vi "RTMain.Close.vi"(11 "cluster":T1 {"Parameters"."Settings"."Data Refs"."Write Refs" format="%.0x"; "Parameters"."Settings"."Data Refs"."Read Refs" format="%.0x"; "Parameters"."Settings"."Write Locations"."DataType" items=["Boolean"=1, "SByte"=2, "Byte"=3, "Int16"=4, "UInt16"=5, "Int32"=6, "UInt32"=7, "Int64"=8, "UInt64"=9, "Float"=10, "Double"=11, "String"=12, "DateTime"=13, "ByteString"=15, "Array of Boolean"=101, "Array of SByte"=102, "Array of Byte"=103, "Array of Int16"=104, "Array of UInt16"=105, "Array of Int32"=106, "Array of UInt32"=107, "Array of Int64"=108, "Array of UInt64"=109, "Array of Float"=110, "Array of Double"=111, "Array of String"=112, "Array of DateTime"=113, "Array of ByteString"=115]}) -> ()   [LabVIEW 2015, in "OPC UA Client Engine.lvlib"]
uses:
  OPC UA Client Engine.lvlib
  Types/Main.StateVariables.ctl
  <vilib>/NI/NIVS Inline Async API/_VS Inline Async API/VS Inline Async API/VS Inline Async API.lvclass
  Types/Poll.Parameters.ctl
  Shared/Compiled.Settings.ctl
  Shared/OPCConnection.Properties.ctl
  Shared/Poll.ListProperties.ctl
  Shared/Tag.WriteProperties.Info.ctl
  Shared/Tags.ReadWriteRefs.ctl
  <vilib>/NI Veristand/Custom Device API/Data Reference.ctl
  <vilib>/NI Veristand/Custom Device API/Custom Device Target Type.ctl
  <vilib>/NI Veristand/Custom Device Tools/Custom Device Utility Library/Custom Device Utility Library.lvlib
  Shared/OPC UA Client Shared.lvlib
  <vilib>/NI VeriStand/Custom Device API/Custom Device API.lvlib
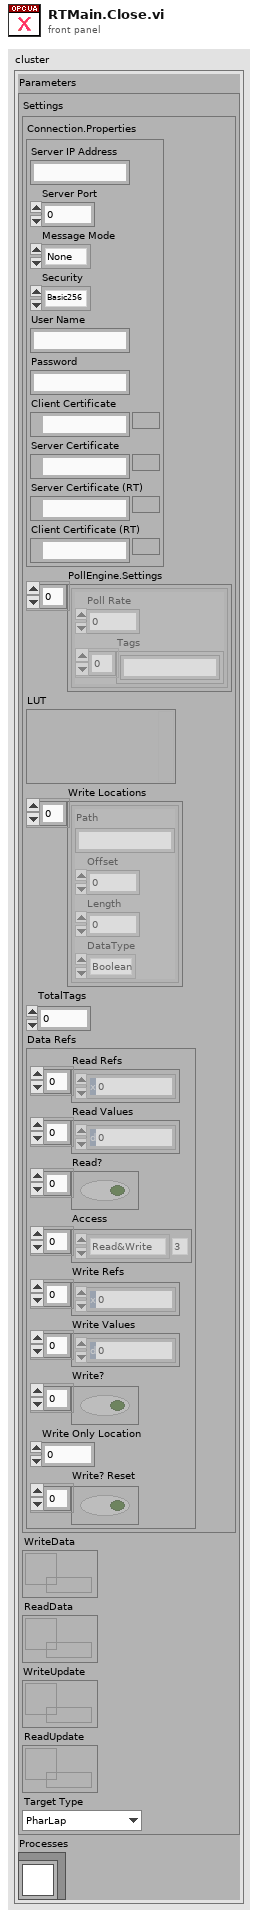
[diagram p1: front panel]
types:
  T1 = typedef "OPC UA Client Engine.lvlib/Main.StateVariables.ctl" = cluster{"Parameters":T2, "Processes":refnum<class "VS Inline Async API.lvclass">}
  T2 = typedef "OPC UA Client Engine.lvlib/Poll.Parameters.ctl" = cluster{"Settings":T3, "WriteData":refnum<k33>, "ReadData":refnum<k33>, "WriteUpdate":refnum<k33>, "ReadUpdate":refnum<k33>, "Target Type":T9}
  T3 = typedef "OPC UA Client Shared.lvlib/Compiled.Settings.ctl" = cluster{"Connection.Properties":T4, "PollEngine.Settings":T5[], "LUT":variant, "Write Locations":T6[], "TotalTags":u32, "Data Refs":T7}
  T4 = typedef "OPC UA Client Shared.lvlib/OPCConnection.Properties.ctl" = cluster{"Server IP Address":string, "Server Port":u16, "Message Mode":enum16{"None", "Sign", "Sign and Encrypt"}, "Security":enum16{"Basic256", "Basic128Rsa15"}, "User Name":string, "Password":string, "Client Certificate":path, "Server Certificate":path, "Server Certificate (RT)":path, "Client Certificate (RT)":path}
  T5 = typedef "OPC UA Client Shared.lvlib/Poll.ListProperties.ctl" = cluster{"Poll Rate":dbl, "Tags":string[]}
  T6 = typedef "OPC UA Client Shared.lvlib/Tag.WriteProperties.Info.ctl" = cluster{"Path":string, "Offset":i32, "Length":i32, "DataType":u32}
  T7 = typedef "OPC UA Client Shared.lvlib/Tags.ReadWriteRefs.ctl" = cluster{"Read Refs":T8[], "Read Values":dbl[], "Read?":bool[], "Access":enum8{"Null", "Read", "Write", "Read&Write"}[], "Write Refs":T8[], "Write Values":dbl[], "Write?":bool[], "Write Only Location":u32, "Write? Reset":bool[]}
  T8 = typedef "Custom Device API.lvlib/Data Reference.ctl" = i32
  T9 = typedef "Custom Device API.lvlib/Custom Device Target Type.ctl" = enum16{"PharLap", "VxWorks", "Windows", "Linux_32_ARM", "Linux_x64"}
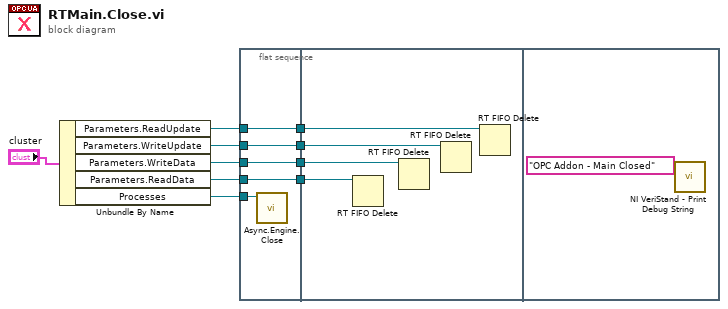
[diagram p0: block diagram]
diagram:
  n1 = Unbundle By Name("cluster") -> ("Parameters.ReadUpdate"=w10:refnum<k33>, "Parameters.WriteUpdate"=w9:refnum<k33>, "Parameters.WriteData"=w8:refnum<k33>, "Parameters.ReadData"=w7:refnum<k33>, "Processes"=w6:refnum<class "VS Inline Async API.lvclass">)
  n2 = flat-sequence {
    tunnel: [w15] -> w4
    tunnel: [w14] -> w3
    tunnel: [w13] -> w2
    tunnel: [w12] -> w1
    tunnel: w6 -> [w11]
    tunnel: w7 -> [w15]
    tunnel: w8 -> [w14]
    tunnel: w9 -> [w13]
    tunnel: w10 -> [w12]
    tunnel: w4 -> [w19]
    tunnel: w3 -> [w18]
    tunnel: w2 -> [w17]
    tunnel: w1 -> [w16]
    frame #0 {
      n3 = call <vilib>:"Async.Engine.Close.vi"("Async in"=w11) -> ()  [unwired: 9 in, 2 out]
    }
    frame #1 {
      n4 = RT FIFO Delete(0:w19) -> ()  [unwired: 2 in, 1 out]
      n5 = RT FIFO Delete(0:w18) -> ()  [unwired: 2 in, 1 out]
      n6 = RT FIFO Delete(0:w17) -> ()  [unwired: 2 in, 1 out]
      n7 = RT FIFO Delete(0:w16) -> ()  [unwired: 2 in, 1 out]
    }
    frame #2 {
      n8 = call <vilib>:"NI VeriStand - Print Debug String.vi"("Message"="OPC Addon - Main Closed") -> ()  [unwired: 10 in, 1 out]
    }
  }
